vi "Write Use Custom CLIP_.vi"(8 "error in (no error)":errorcluster, 10 "Use Custom CLIP?":bool, 11 "RIO Target Configuration in":refnum<class "RIO Target Configuration.lvclass">) -> (0 "error out":errorcluster, 3 "RIO Target Configuration out":refnum<class "RIO Target Configuration.lvclass">)   [LabVIEW 2014, in "RIO Target Configuration.lvclass"]
uses:
  RIO Target Configuration.lvclass
  RIO Target Configuration.lvclass/RIO Target Configuration.ctl
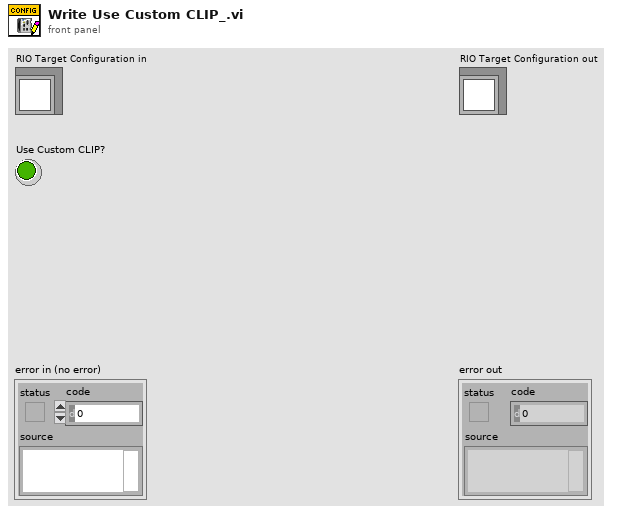
[diagram p1: front panel]
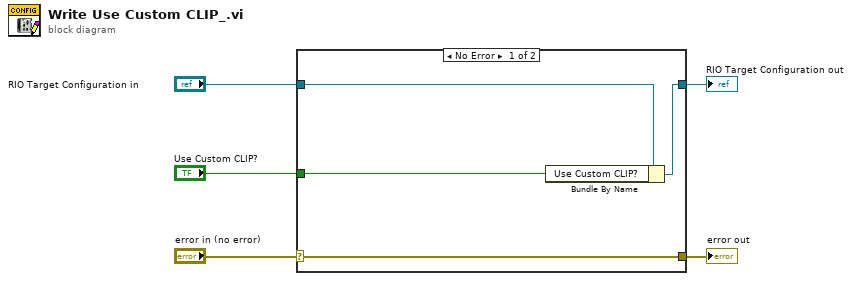
[diagram p0: block diagram]
diagram:
  n1 = case shown="No Error" "error in (no error)" {
    selector: "error in (no error)" -> [w9 w10]
    tunnel: [w9 w10] -> w4
    tunnel: [w7 w11] -> w2
    tunnel: "RIO Target Configuration in" -> [w8 w11]
    tunnel: "Use Custom CLIP?" -> [w6 _]
    frame No Error {
      n2 = Bundle By Name(cluster=w8, "Use Custom CLIP?"=w6) -> (w7:refnum<class "RIO Target Configuration.lvclass">)
    }
    frame Error {
    }
  }
  "error out" <- w4
  "RIO Target Configuration out" <- w2
